vi "clear all.vi"   [LabVIEW 2023]
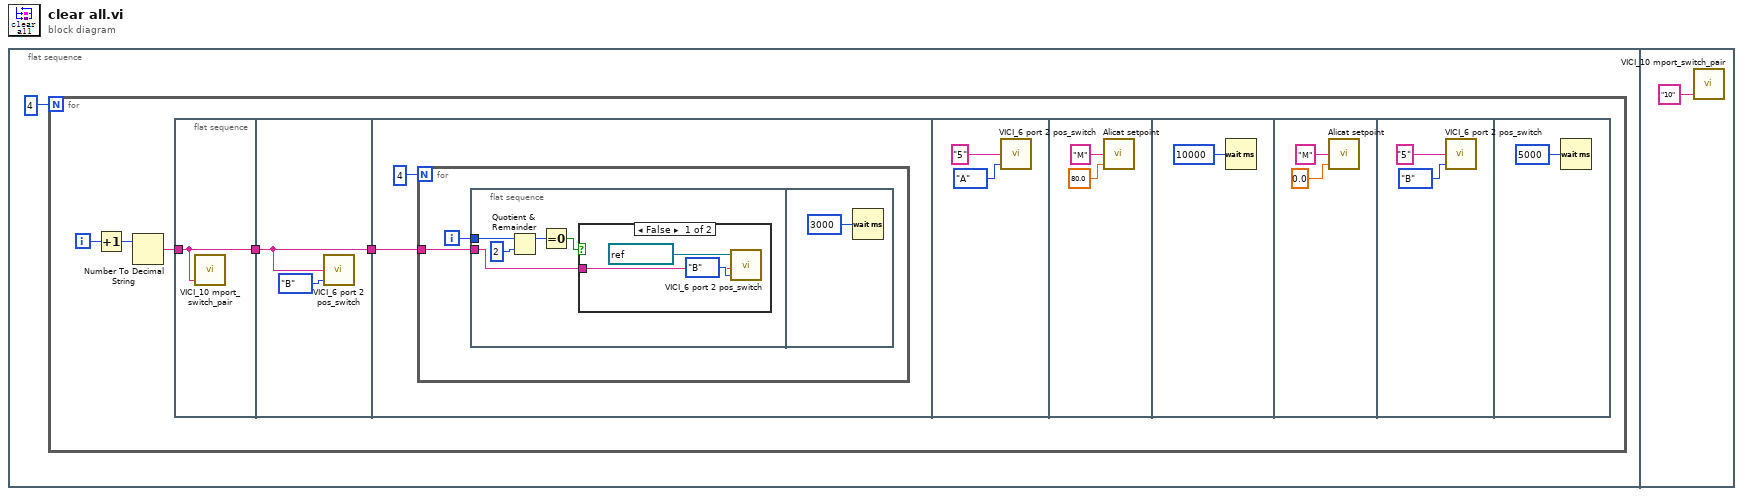
[diagram p0: block diagram]
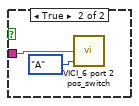
[diagram p2: hidden frame]
diagram:
  n1 = flat-sequence {
    frame #0 {
      n2 = for {
        N: 4 -> [_]
        i -> [w6]
        n3 = Increment(x=w6) -> (x+1=w5:i32)
        n4 = Number To Decimal String(number=w5) -> (decimal integer string=w4:string)  [unwired: 1 in]
        n5 = flat-sequence {
          tunnel: w4 -> [w7]
          tunnel: [w7] -> w3
          tunnel: w3 -> [w8]
          tunnel: [w8] -> w2
          tunnel: w2 -> [w10]
          frame #0 {
            n6 = call "VICI_10 mport_switch_pair.vi"("Go to position"=w7) -> ()  [unwired: 3 in, 1 out]
          }
          frame #1 {
            n7 = call "VICI_6 port 2 pos_switch.vi"("Switch to position (A/B)"=enum16{"A", "B"}."B", "Valve ID"=w8) -> ()  [unwired: 2 in, 1 out]
          }
          frame #2 {
            n8 = for {
              N: 4 -> [_]
              tunnel: w10 -> [w12]
              i -> [w13]
              n9 = flat-sequence {
                tunnel: w13 -> [w18]
                tunnel: w12 -> [w14]
                frame #0 {
                  n10 = Quotient & Remainder(x=w18, y=2) -> (x-y*floor(x/y)=w16:i32)  [unwired: 1 out]
                  n11 = Equal To 0?(x=w16) -> (x = 0?=w15:bool)
                  n12 = case shown="False" w15 {
                    tunnel: w14 -> [w19 w22]
                    frame False {
                      n13 = call "VICI_6 port 2 pos_switch.vi"("Switch to position (A/B)"=enum16{"A", "B"}."B", "Valve ID"=w19, "Valve COM"=refnum<visa-resource-name> "COM8") -> ()  [unwired: 1 in, 1 out]
                    }
                    frame True {
                      n14 = call "VICI_6 port 2 pos_switch.vi"("Switch to position (A/B)"=enum16{"A", "B"}."A", "Valve ID"=w22) -> ()  [unwired: 2 in, 1 out]
                    }
                  }
                }
                frame #1 {
                  n15 = Wait (ms)(milliseconds to wait=u32 3000) -> ()  [unwired: 1 out]
                }
              }
            }
          }
          frame #3 {
            n16 = call "VICI_6 port 2 pos_switch.vi"("Switch to position (A/B)"=enum16{"A", "B"}."A", "Valve ID"="5") -> ()  [unwired: 2 in, 1 out]
          }
          frame #4 {
            n17 = call "Alicat setpoint.vi"("Setpoint"=80.0, "Unit ID"="M") -> ()  [unwired: 3 in]
          }
          frame #5 {
            n18 = Wait (ms)(milliseconds to wait=u32 10000) -> ()  [unwired: 1 out]
          }
          frame #6 {
            n19 = call "Alicat setpoint.vi"("Setpoint"=0.0, "Unit ID"="M") -> ()  [unwired: 3 in]
          }
          frame #7 {
            n20 = call "VICI_6 port 2 pos_switch.vi"("Switch to position (A/B)"=enum16{"A", "B"}."B", "Valve ID"="5") -> ()  [unwired: 2 in, 1 out]
          }
          frame #8 {
            n21 = Wait (ms)(milliseconds to wait=u32 5000) -> ()  [unwired: 1 out]
          }
        }
      }
    }
    frame #1 {
      n22 = call "VICI_10 mport_switch_pair.vi"("Go to position"="10") -> ()  [unwired: 3 in, 1 out]
    }
  }
